vi "ClassName.vi"(8 "error in (no error)":errorcluster, 11 "Class 2 in":refnum<class "Class 2.lvclass">) -> (0 "error out":errorcluster, 2 "ClassName":string, 3 "Class 2 out":refnum<class "Class 2.lvclass">)   [LabVIEW 2021, in "Class 2.lvclass"]
uses:
  Class 2.lvclass
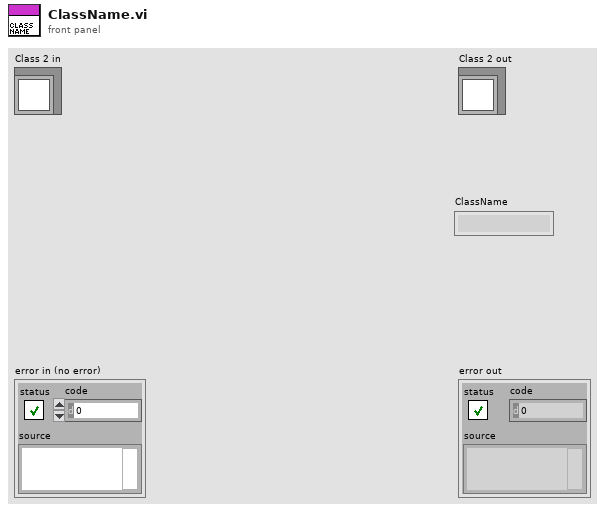
[diagram p1: front panel]
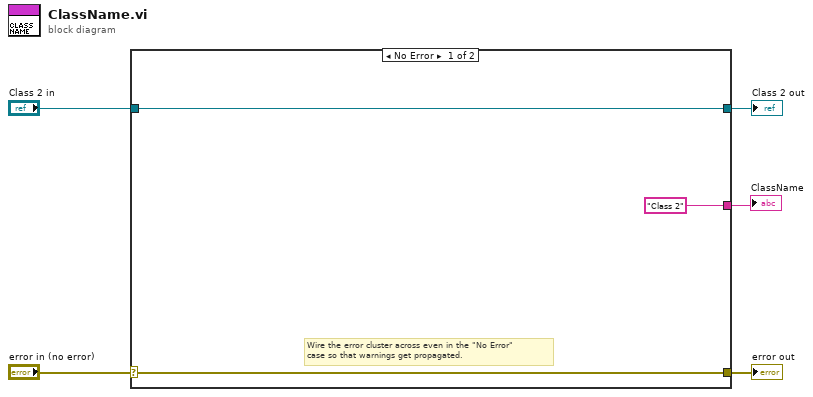
[diagram p0: block diagram]
diagram:
  n1 = case shown="No Error" "error in (no error)" {
    selector: "error in (no error)" -> [w7 w10]
    tunnel: [w7 w10] -> w4
    tunnel: [w8 w9] -> w2
    tunnel: "Class 2 in" -> [w8 w9]
    tunnel: ["Class 2" ("ClassName") _] -> w1
    frame No Error {
      # "Wire the error cluster across even in the \"No Error\"\ncase so that warnings get propagated."
    }
    frame Error {
    }
  }
  "error out" <- w4
  "Class 2 out" <- w2
  "ClassName" <- w1
